vi "trim image.vi"(10 "scale":i32=2, 11 "Image Pixels (U32)":u32[][](array[numeric])) -> (3 "Trimmed Image Pixels (U32)":u32[][](array[numeric]))   [LabVIEW 2017]
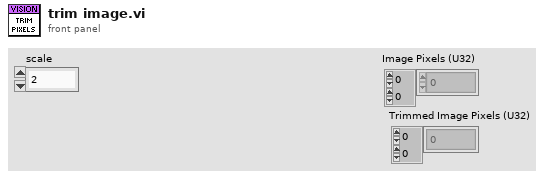
[diagram p1: front panel]
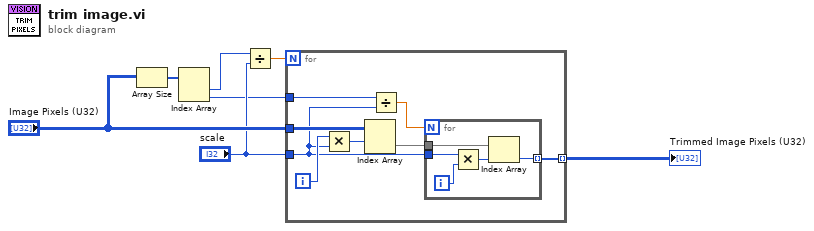
[diagram p0: block diagram]
diagram:
  n1 = Array Size(array="Image Pixels (U32)") -> (size(s)=w6:i32[])
  n2 = Index Array(array=w6) -> (element #1=w4:i32, element #2=w2:i32)  [unwired: 2 in]
  n3 = Divide(x=w4, y="scale") -> (x/y=w5:dbl)
  n4 = for {
    N: w5 -> [_]
    tunnel: "Image Pixels (U32)" -> [w15]
    tunnel: "scale" -> [w9]
    tunnel: w2 -> [w10]
    tunnel: [w8] -> w1 mode=indexing
    i -> [w14]
    n5 = Multiply(x=w14, y=w9) -> (x*y=w13:i32)
    n6 = Index Array(array=w15, index (row)=w13) -> (element=w12:u32[])  [unwired: 1 in]
    n7 = Divide(x=w10, y=w9) -> (x/y=w11:dbl)
    n8 = for {
      N: w11 -> [_]
      tunnel: w12 -> [w20]
      tunnel: w9 -> [w18]
      tunnel: [w16] -> w8 mode=indexing
      i -> [w17]
      n9 = Multiply(x=w18, y=w17) -> (x*y=w19:i32)
      n10 = Index Array(array=w20, index=w19) -> (element=w16:u32)
    }
  }
  "Trimmed Image Pixels (U32)" <- w1
